vi "FT10_Semi-Auto Parse Commands.vi"(11 "Semi-Auto Cluster":T2) -> (3 "appended array":T1[](array[typedef]))   [LabVIEW 2015]
uses:
  Controls/Control_Semi-Auto Cluster.ctl
  Controls/Control_Semi-Auto Unitherm Load.ctl
  Controls/Control_Semi-Auto Port.ctl
  Controls/Control_Semi-Auto Mode.ctl
  Controls/Control_Semi-Auto Power Level.ctl
  Controls/Control_Semi-Auto Activation Duration.ctl
  Controls/Control_Command Cluster.ctl
  Controls/Control_Fornax Mono2 Cut Enum.ctl
  Controls/Control_Fornax Mono2 Coag Enum.ctl
  Controls/Control_Fornax Mono1 Cut Enum.ctl
  Controls/Control_Fornax Mono1 Coag Enum.ctl
  Controls/Control_Fornax Bipolar Enum.ctl
  Controls/Control_Fornax Ligasure Activate Port Bool.ctl
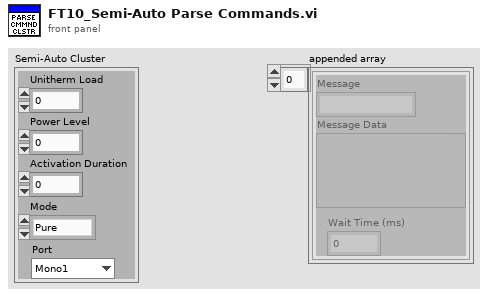
[diagram p1: front panel]
types:
  T1 = typedef "Control_Command Cluster.ctl" = cluster{"Message":string, "Message Data":variant, "Wait Time (ms)":i32}
  T2 = typedef "Control_Semi-Auto Cluster.ctl" = cluster{"Unitherm Load":T3, "Port":T4, "Mode":T5, "Power Level":T6, "Activation Duration":T7}
  T3 = typedef "Control_Semi-Auto Unitherm Load.ctl" = i32
  T4 = typedef "Control_Semi-Auto Port.ctl" = enum16{"Mono1", "Mono2", "Bipolar", "Ligasure", "Error"}
  T5 = typedef "Control_Semi-Auto Mode.ctl" = enum16{"Pure", "Blend", "Spray", "Fulgerate", "Standard", "Macro", "Precision", "Ligasure", "Error"}
  T6 = typedef "Control_Semi-Auto Power Level.ctl" = i32
  T7 = typedef "Control_Semi-Auto Activation Duration.ctl" = i32
  T8 = typedef "Control_Fornax Ligasure Activate Port Bool.ctl" = bool
  T9 = typedef "Control_Fornax Mono2 Cut Enum.ctl" = enum16{"Pure", "Blend"}
  T10 = typedef "Control_Fornax Mono2 Coag Enum.ctl" = enum16{"Fulgerate", "Spray"}
  T11 = typedef "Control_Fornax Mono1 Cut Enum.ctl" = enum16{"Pure", "Blend"}
  T12 = typedef "Control_Fornax Mono1 Coag Enum.ctl" = enum16{"Fulgerate", "Spray"}
  T13 = typedef "Control_Fornax Bipolar Enum.ctl" = enum16{"Standard", "Macro", "Precision"}
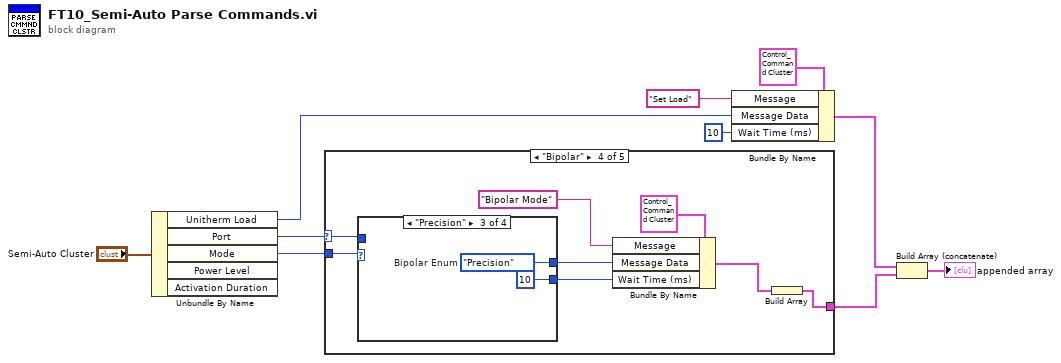
[diagram p0: block diagram]
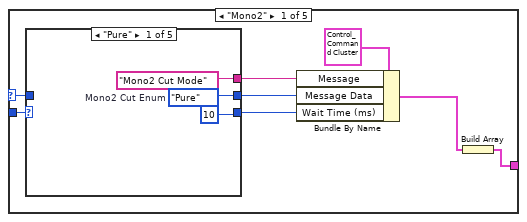
[diagram p2: hidden frame]
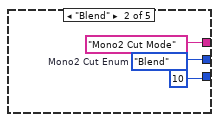
[diagram p3: hidden frame]
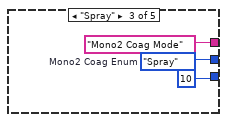
[diagram p4: hidden frame]
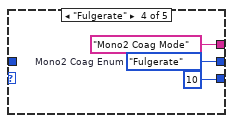
[diagram p5: hidden frame]
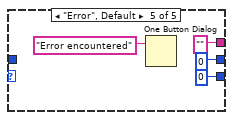
[diagram p6: hidden frame]
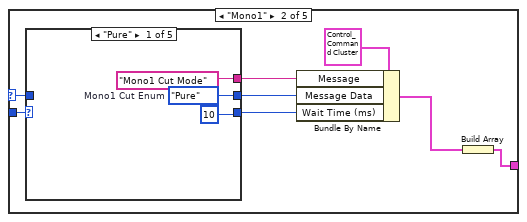
[diagram p7: hidden frame]
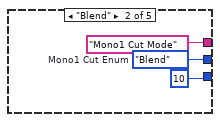
[diagram p8: hidden frame]
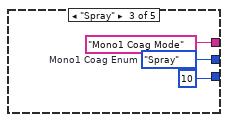
[diagram p9: hidden frame]
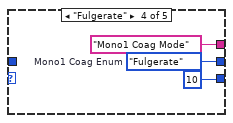
[diagram p10: hidden frame]
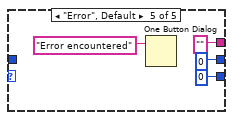
[diagram p11: hidden frame]
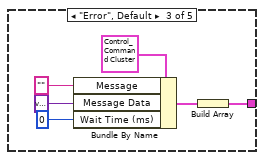
[diagram p12: hidden frame]
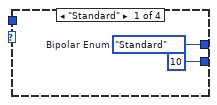
[diagram p13: hidden frame]
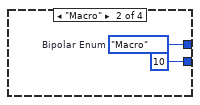
[diagram p14: hidden frame]
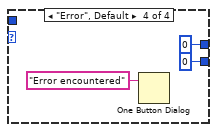
[diagram p15: hidden frame]
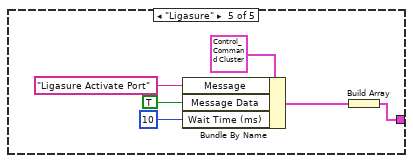
[diagram p16: hidden frame]
diagram:
  n1 = Unbundle By Name("Semi-Auto Cluster") -> ("Unitherm Load"=w6:T3, "Port"=w3:T4, "Mode"=w2:T5)  [unwired: 2 out]
  n2 = case shown="\"Bipolar\"" w3 {
    selector: w3 -> [w17 w41 _ w71 _]
    tunnel: w2 -> [w18 w42 _ w72 _]
    tunnel: [w11 w35 w62 w65 w85] -> w1
    frame "Mono2" {
      n3 = case shown="\"Pure\"" w18 {
        tunnel: w17 -> [_ _ _ _ _]
        tunnel: [w21 w24 w27 w30 u16 0 ("Mono2 Coag Enum")] -> w14
        tunnel: ["Mono2 Cut Mode" ("Message") "Mono2 Cut Mode" ("Message") "Mono2 Coag Mode" ("Message") "Mono2 Coag Mode" ("Message") "" ("Message")] -> w15
        tunnel: [10 ("Wait Time (ms)") 10 ("Wait Time (ms)") 10 ("Wait Time (ms)") 10 ("Wait Time (ms)") 0 ("Wait Time (ms)")] -> w13
        frame "Pure" {
          w21 = Control_Fornax_Mono2_Cut_Enum."Pure"  # Mono2 Cut Enum
        }
        frame "Blend" {
          w24 = Control_Fornax_Mono2_Cut_Enum."Blend"  # Mono2 Cut Enum
        }
        frame "Spray" {
          w27 = Control_Fornax_Mono2_Coag_Enum."Spray"  # Mono2 Coag Enum
        }
        frame "Fulgerate" {
          w30 = Control_Fornax_Mono2_Coag_Enum."Fulgerate"  # Mono2 Coag Enum
        }
        frame "Error", Default {
          n4 = One Button Dialog(message="Error encountered") -> ()  [unwired: 1 in, 1 out]
        }
      }
      n5 = Bundle By Name(cluster=T1 {"Message"="", "Message Data"=variant, "Wait Time (ms)"=0}, "Message"=w15, "Message Data"=w14, "Wait Time (ms)"=w13) -> (w12:T1)
      n6 = Build Array(w12) -> (w11:T1[])
    }
    frame "Mono1" {
      n7 = case shown="\"Pure\"" w42 {
        tunnel: w41 -> [_ _ _ _ _]
        tunnel: [w43 w46 w49 w52 u16 0 ("Mono2 Coag Enum")] -> w38
        tunnel: ["Mono1 Cut Mode" ("Message") "Mono1 Cut Mode" ("Message") "Mono1 Coag Mode" ("Message") "Mono1 Coag Mode" ("Message") "" ("Message")] -> w39
        tunnel: [10 ("Wait Time (ms)") 10 ("Wait Time (ms)") 10 ("Wait Time (ms)") 10 ("Wait Time (ms)") 0 ("Wait Time (ms)")] -> w37
        frame "Pure" {
          w43 = Control_Fornax_Mono1_Cut_Enum."Pure"  # Mono1 Cut Enum
        }
        frame "Blend" {
          w46 = Control_Fornax_Mono1_Cut_Enum."Blend"  # Mono1 Cut Enum
        }
        frame "Spray" {
          w49 = Control_Fornax_Mono1_Coag_Enum."Spray"  # Mono1 Coag Enum
        }
        frame "Fulgerate" {
          w52 = Control_Fornax_Mono1_Coag_Enum."Fulgerate"  # Mono1 Coag Enum
        }
        frame "Error", Default {
          n8 = One Button Dialog(message="Error encountered") -> ()  [unwired: 1 in, 1 out]
        }
      }
      n9 = Bundle By Name(cluster=T1 {"Message"="", "Message Data"=variant, "Wait Time (ms)"=0}, "Message"=w39, "Message Data"=w38, "Wait Time (ms)"=w37) -> (w36:T1)
      n10 = Build Array(w36) -> (w35:T1[])
    }
    frame "Error", Default {
      n11 = Bundle By Name(cluster=T1 {"Message"="", "Message Data"=variant, "Wait Time (ms)"=0}, "Message"="", "Message Data"=variant, "Wait Time (ms)"=0) -> (w63:T1)
      n12 = Build Array(w63) -> (w62:T1[])
    }
    frame "Bipolar" {
      n13 = case shown="\"Precision\"" w72 {
        tunnel: w71 -> [_ _ _ _]
        tunnel: [w74 w76 w78 u16 0 ("Mono2 Coag Enum")] -> w68
        tunnel: [10 ("Wait Time (ms)") 10 ("Wait Time (ms)") 10 ("Wait Time (ms)") 0 ("Wait Time (ms)")] -> w67
        frame "Standard" {
          w74 = Control_Fornax_Bipolar_Enum."Standard"  # Bipolar Enum
        }
        frame "Macro" {
          w76 = Control_Fornax_Bipolar_Enum."Macro"  # Bipolar Enum
        }
        frame "Precision" {
          w78 = Control_Fornax_Bipolar_Enum."Precision"  # Bipolar Enum
        }
        frame "Error", Default {
          n14 = One Button Dialog(message="Error encountered") -> ()  [unwired: 1 in, 1 out]
        }
      }
      n15 = Bundle By Name(cluster=T1 {"Message"="", "Message Data"=variant, "Wait Time (ms)"=0}, "Message"="Bipolar Mode", "Message Data"=w68, "Wait Time (ms)"=w67) -> (w66:T1)
      n16 = Build Array(w66) -> (w65:T1[])
    }
    frame "Ligasure" {
      n17 = Bundle By Name(cluster=T1 {"Message"="", "Message Data"=variant, "Wait Time (ms)"=0}, "Message"="Ligasure Activate Port", "Message Data"=T8 TRUE ("Ligasure Activate"), "Wait Time (ms)"=10) -> (w84:T1)
      n18 = Build Array(w84) -> (w85:T1[])
    }
  }
  n19 = Bundle By Name(cluster=T1 {"Message"="", "Message Data"=variant, "Wait Time (ms)"=0}, "Message"="Set Load", "Message Data"=w6, "Wait Time (ms)"=10) -> (w9:T1)
  n20 = Build Array (concatenate)(w9, w1) -> (→"appended array":T1[])
